vi "building metadata array.vi"() -> ()   [LabVIEW 2013]
panel:
  out "custom metadata array":T1(array[cluster])
  in  "extra information field":T2={"Attribute"="", "Value"="", "Data type"=enum."<null>"}
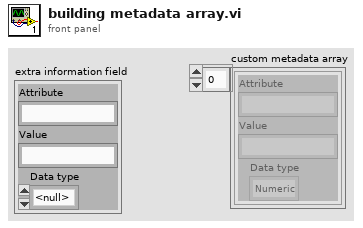
[diagram p1: front panel]
types:
  T1 = cluster{"Attribute":string, "Value":string, "Data type":enum16{"Numeric", "String", "1D array of strings", "1D array of doubles", "Data JSON string", "<null>"}}[]
  T2 = cluster{"Attribute":string, "Value":string, "Data type":enum16{"Numeric", "String", "1D array of strings", "1D array of doubles", "Data JSON string", "<null>"}}
  T3 = enum16{"Numeric", "String", "1D array of strings", "1D array of doubles", "Data JSON string", "<null>"}
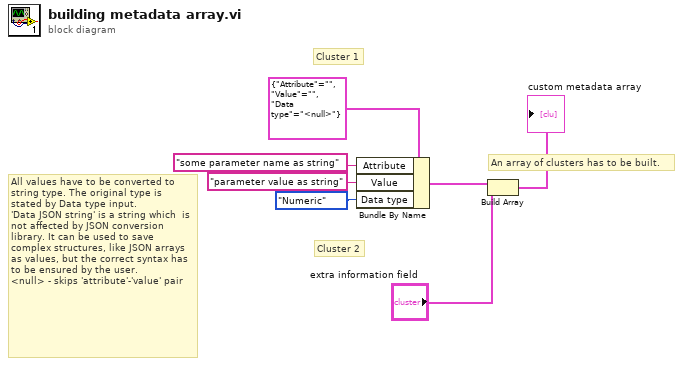
[diagram p0: block diagram]
diagram:
  # "An array of clusters has to be built."
  # "Cluster 2"
  # "Cluster 1"
  # "All values have to be converted to string type. The original type is stated by Data type input.\n'Data JSON string' is a string which  is not affected by JSON conversion library. It can be used to save complex structures, like JSON arrays as values, but the correct syntax has  to be ensured by the user.\n<null> - skips 'attribute'-'value' pair"
  n1 = Bundle By Name(cluster=T2 {"Attribute"="", "Value"="", "Data type"=enum."<null>"} ("extra information field 4"), "Attribute"="some parameter name as string", "Value"="parameter value as string", "Data type"=T3."Numeric") -> (w3:T2)
  n2 = Build Array(w3, "extra information field") -> (→"custom metadata array":T1)
